vi "make_buttons_available.vi"(0 "array":refnum<vi>[](array[refnum]), 1 "Make Available":bool) -> ()   [LabVIEW 2015]
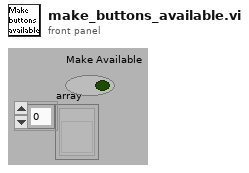
[diagram p1: front panel]
types:
  T1 = cluster{"array[0]":refnum<vi>, "array[1]":refnum<vi>, "array[2]":refnum<vi>, "array[3]":refnum<vi>, "array[4]":refnum<vi>, "array[5]":refnum<vi>}
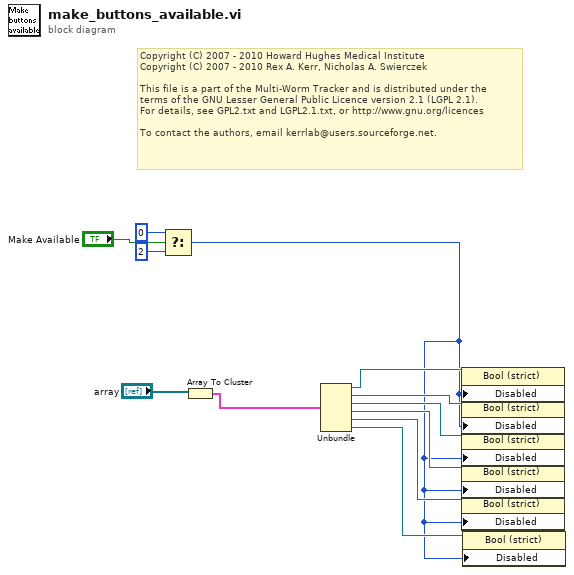
[diagram p0: block diagram]
diagram:
  # "Copyright (C) 2007 - 2010 Howard Hughes Medical Institute\nCopyright (C) 2007 - 2010 Rex A. Kerr, Nicholas A. Swierczek\n \nThis file is a part of the Multi-Worm Tracker and is distributed under the\nterms of the GNU Lesser General Public Licence version 2.1 (LGPL 2.1).\nFor details, see GPL2.txt and LGPL2.1.txt, or http://www.gnu.org/licences\n \nTo contact the authors, email kerrlab@users.sourceforge.net."
  n1 = Select(t=0, s="Make Available", f=2) -> (s? t:f=w1:i32)
  n2 = Array To Cluster(array="array") -> (cluster=w7:T1)
  n3 = Unbundle(w7) -> ("array[0]"=w12:refnum<vi>, "array[1]"=w11:refnum<vi>, "array[2]"=w10:refnum<vi>, "array[3]"=w9:refnum<vi>, "array[4]"=w8:refnum<vi>, "array[5]"=w5:refnum<vi>)
  n4 = property class="Bool (strict)"(reference=w12, "Disabled"=w1) -> ()  [unwired: 1 in, 2 out]
  n5 = property class="Bool (strict)"(reference=w11, "Disabled"=w1) -> ()  [unwired: 1 in, 2 out]
  n6 = property class="Bool (strict)"(reference=w10, "Disabled"=w1) -> ()  [unwired: 1 in, 2 out]
  n7 = property class="Bool (strict)"(reference=w9, "Disabled"=w1) -> ()  [unwired: 1 in, 2 out]
  n8 = property class="Bool (strict)"(reference=w8, "Disabled"=w1) -> ()  [unwired: 1 in, 2 out]
  n9 = property class="Bool (strict)"(reference=w5, "Disabled"=w1) -> ()  [unwired: 1 in, 2 out]
